vi "RSZVB Get Trace Smoothing.vi"(8 "error in (no error)":errorcluster {"code" format="%.0x"}, 10 "Channel (Trace) (1)":i32=1, 11 "VISA session":refnum<visa-resource-name>) -> (0 "error out":errorcluster {"code" format="%.0x"}, 1 "Smoothing":bool, 2 "Aperture":dbl format="%^.3e", 3 "dup VISA session":refnum<visa-resource-name>)   [LabVIEW 2011]
doc: "This VI returns state of the smoothing VI parameters.\n\nRemote-control command(s):\nCALCulate<Ch/Tr>:SMOothing[:STATe]?\nCALCulate<Ch/Tr>:SMOothing:APERture?"
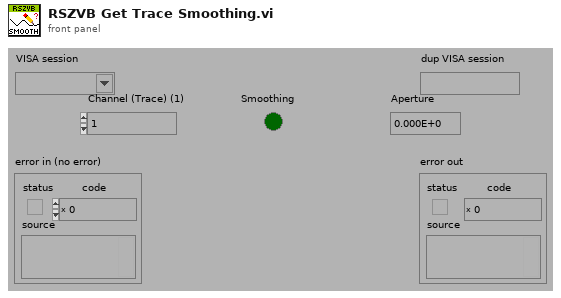
[diagram p1: front panel]
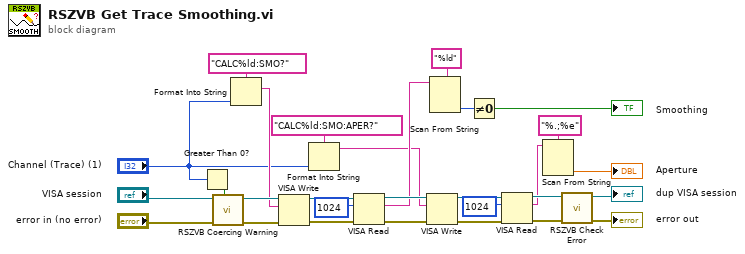
[diagram p0: block diagram]
diagram:
  n1 = Greater Than 0?(x="Channel (Trace) (1)") -> (x > 0?=w20:bool)
  n2 = call "RSZVB Coercing Warning.vi"("In Range?"=w20, "error in (no error)"="error in (no error)", "VISA session"="VISA session") -> ("error out"=w27:errorcluster, "dup VISA session"=w28:refnum<visa-resource-name>)  [unwired: 7 in]
  n3 = Format Into String(format string="CALC%ld:SMO?", "Channel (Trace) (1)") -> (resulting string=w26:string)  [unwired: 2 in, 1 out]
  n4 = VISA Write(VISA resource name=w28, write buffer=w26, error in (no error)=w27) -> (VISA resource name out=w23:refnum<visa-resource-name>, error out=w24:errorcluster)  [unwired: 1 out]
  n5 = Format Into String(format string="CALC%ld:SMO:APER?", "Channel (Trace) (1)") -> (resulting string=w2:string)  [unwired: 2 in, 1 out]
  n6 = VISA Read(VISA resource name=w23, byte count=u32 1024 ("byte count (0)"), error in (no error)=w24) -> (VISA resource name out=w15:refnum<visa-resource-name>, read buffer=w5:string, error out=w14:errorcluster)  [unwired: 1 out]
  n7 = VISA Write(VISA resource name=w15, write buffer=w2, error in (no error)=w14) -> (VISA resource name out=w19:refnum<visa-resource-name>, error out=w13:errorcluster)  [unwired: 1 out]
  n8 = Scan From String(format string="%ld", input string=w5) -> (output 1=w6:i32)  [unwired: 3 in, 3 out]
  n9 = Not Equal To 0?(x=w6) -> (x != 0?=→"Smoothing":bool)
  n10 = VISA Read(VISA resource name=w19, byte count=u32 1024 ("byte count (0)"), error in (no error)=w13) -> (VISA resource name out=w16:refnum<visa-resource-name>, read buffer=w9:string, error out=w17:errorcluster)  [unwired: 1 out]
  n11 = Scan From String(format string="%.;%e", input string=w9) -> (output 1=→"Aperture":dbl)  [unwired: 3 in, 3 out]
  n12 = call "RSZVB Check Error.vi"("error in (no error)"=w17, "VISA session"=w16) -> ("error out"=→"error out":errorcluster, "dup VISA session"=→"dup VISA session":refnum<visa-resource-name>)  [unwired: 8 in]
